vi "Recipe_Line_Update_Sub1.vi"(11 "Parameters":T1) -> (3 "Parameter_str":string[](array[string]))   [LabVIEW 2014]
panel:
  out "Operation_Mode":enum16{"PinSweep", "SingleMeasure"}(ring)
  out "Standard":enum16{"CW", "LTE", "WCDMA", "GSM", "EDGE"}(ring)
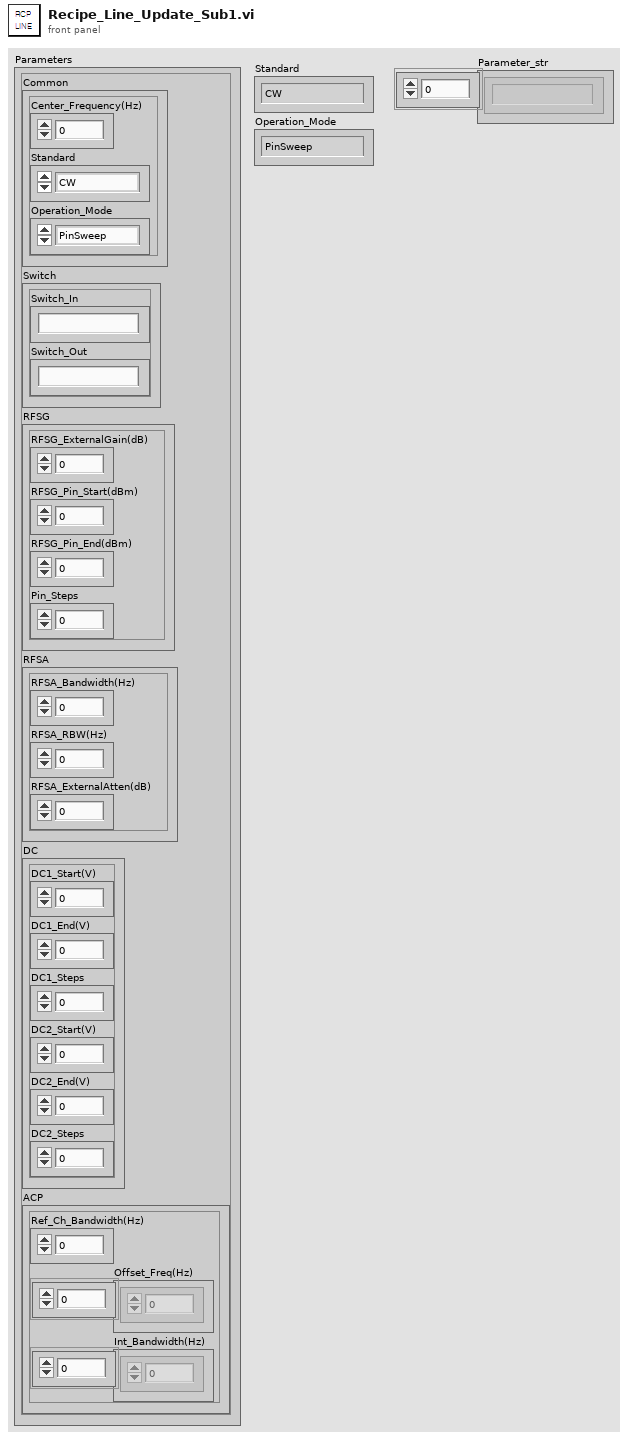
[diagram p1: front panel]
types:
  T1 = cluster{"Common":cluster{"Center_Frequency(Hz)":dbl, "Standard":enum16{"CW", "LTE", "WCDMA", "GSM", "EDGE"}, "Operation_Mode":enum16{"PinSweep", "SingleMeasure"}}, "Switch":cluster{"Switch_In":string, "Switch_Out":string}, "RFSG":cluster{"RFSG_ExternalGain(dB)":dbl, "RFSG_Pin_Start(dBm)":dbl, "RFSG_Pin_End(dBm)":dbl, "Pin_Steps":dbl}, "RFSA":cluster{"RFSA_Bandwidth(Hz)":dbl, "RFSA_RBW(Hz)":dbl, "RFSA_ExternalAtten(dB)":dbl}, "DC":cluster{"DC1_Start(V)":dbl, "DC1_End(V)":dbl, "DC1_Steps":dbl, "DC2_Start(V)":dbl, "DC2_End(V)":dbl, "DC2_Steps":dbl}, "ACP":cluster{"Ref_Ch_Bandwidth(Hz)":dbl, "Offset_Freq(Hz)":dbl[], "Int_Bandwidth(Hz)":dbl[]}}
  T2 = cluster{"Center_Frequency(Hz)":dbl, "Standard":enum16{"CW", "LTE", "WCDMA", "GSM", "EDGE"}, "Operation_Mode":enum16{"PinSweep", "SingleMeasure"}}
  T3 = cluster{"RFSG_ExternalGain(dB)":dbl, "RFSG_Pin_Start(dBm)":dbl, "RFSG_Pin_End(dBm)":dbl, "Pin_Steps":dbl}
  T4 = cluster{"RFSA_Bandwidth(Hz)":dbl, "RFSA_RBW(Hz)":dbl, "RFSA_ExternalAtten(dB)":dbl}
  T5 = cluster{"DC1_Start(V)":dbl, "DC1_End(V)":dbl, "DC1_Steps":dbl, "DC2_Start(V)":dbl, "DC2_End(V)":dbl, "DC2_Steps":dbl}
  T6 = cluster{"Ref_Ch_Bandwidth(Hz)":dbl, "Offset_Freq(Hz)":dbl[], "Int_Bandwidth(Hz)":dbl[]}
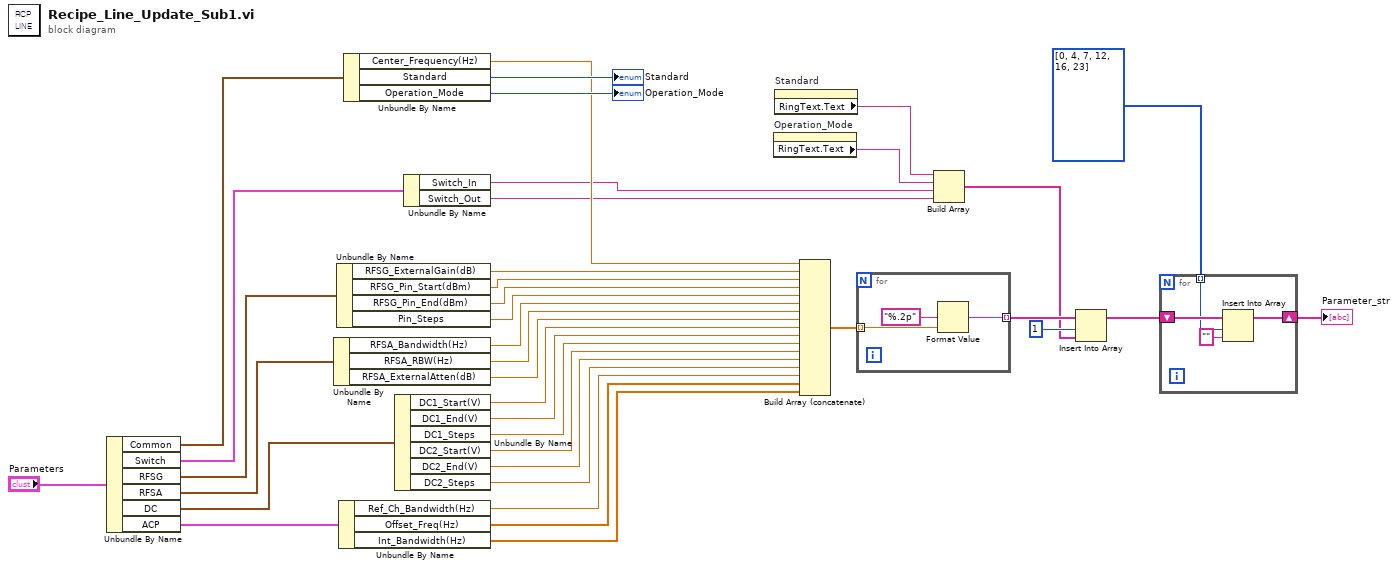
[diagram p0: block diagram]
diagram:
  n1 = Unbundle By Name("Parameters") -> ("Common"=w36:T2, "Switch"=w35:cluster{"Switch_In":string, "Switch_Out":string}, "RFSG"=w34:T3, "RFSA"=w33:T4, "DC"=w32:T5, "ACP"=w31:T6)
  n2 = Unbundle By Name(w33) -> ("RFSA_Bandwidth(Hz)"=w23:dbl, "RFSA_RBW(Hz)"=w22:dbl, "RFSA_ExternalAtten(dB)"=w21:dbl)
  n3 = Unbundle By Name(w34) -> ("RFSG_ExternalGain(dB)"=w27:dbl, "RFSG_Pin_Start(dBm)"=w26:dbl, "RFSG_Pin_End(dBm)"=w25:dbl, "Pin_Steps"=w24:dbl)
  n4 = Unbundle By Name(w31) -> ("Ref_Ch_Bandwidth(Hz)"=w14:dbl, "Offset_Freq(Hz)"=w13:dbl[], "Int_Bandwidth(Hz)"=w12:dbl[])
  n5 = Unbundle By Name(w36) -> ("Center_Frequency(Hz)"=w28:dbl, "Standard"=→"Standard":enum16{"CW", "LTE", "WCDMA", "GSM", "EDGE"}, "Operation_Mode"=→"Operation_Mode":enum16{"PinSweep", "SingleMeasure"})
  n6 = Unbundle By Name(w32) -> ("DC1_Start(V)"=w20:dbl, "DC1_End(V)"=w19:dbl, "DC1_Steps"=w18:dbl, "DC2_Start(V)"=w17:dbl, "DC2_End(V)"=w16:dbl, "DC2_Steps"=w15:dbl)
  n7 = Unbundle By Name(w35) -> ("Switch_In"=w8:string, "Switch_Out"=w9:string)
  n8 = property on="Operation_Mode" class="Enum (strict)"() -> ("RingText.Text"=w7:string)  [unwired: 2 in, 2 out]
  n9 = property on="Standard" class="Enum (strict)"() -> ("RingText.Text"=w10:string)  [unwired: 2 in, 2 out]
  n10 = Build Array (concatenate)(w28, w27, w26, w25, w24, w23, w22, w21, w20, w19, w18, w17, w16, w15, w14, w13, w12) -> (w11:dbl[])
  n11 = for {
    tunnel: w11 -> [w39] mode=indexing
    tunnel: [w38] -> w6 mode=indexing
    n12 = Format Value(format string="%.2p", value (0)=w39) -> (output string=w38:string)  [unwired: 1 in]
  }
  n13 = Build Array(w10, w7, w8, w9) -> (w4:string[])
  n14 = Insert Into Array(array=w6, index=1, new element=w4) -> (w3:string[])
  n15 = for {
    shift-right: [w41] -> w1
    shift-left: w3 -> [w44]
    tunnel: i32[] [0, 4, 7, 12, 16, 23] -> [w43] mode=indexing
    n16 = Insert Into Array(array=w44, index=w43, new element="" ("new element/subarray")) -> (w41:string[])
  }
  "Parameter_str" <- w1
